vi "Generator PBP.vi"(6 "Faza":dbl, 7 "Numeric":dbl, 8 "Offset":dbl, 9 "Czestotliwosc":dbl, 10 "Amplituda":dbl, 11 "Sygnal":T1(ring)) -> (3 "Wyjscie":dbl)   [LabVIEW 2019]
uses:
  <vilib>/ptbypt/NI_PtbyPt.lvlib
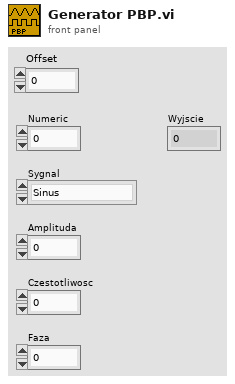
[diagram p1: front panel]
types:
  T1 = enum16{"Sinus", "Prostokąt", "Piła", "Trójkąt", "Rozkład losowy", "Rozkład normalny"}
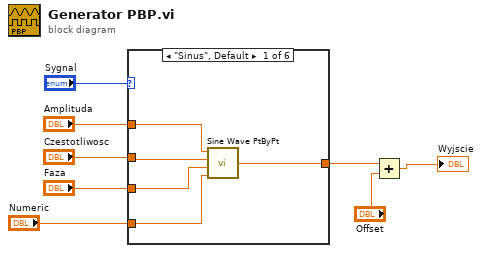
[diagram p0: block diagram]
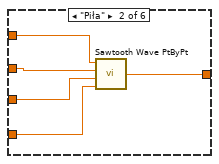
[diagram p2: hidden frame]
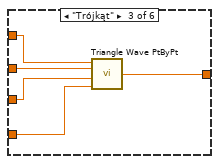
[diagram p3: hidden frame]
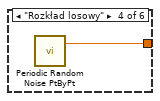
[diagram p4: hidden frame]
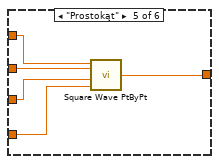
[diagram p5: hidden frame]
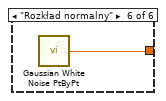
[diagram p6: hidden frame]
diagram:
  n1 = case shown="\"Sinus\", Default" "Sygnal" {
    tunnel: "Amplituda" -> [w13 w15 w19 _ w25 _]
    tunnel: "Czestotliwosc" -> [w12 w16 w20 _ w26 _]
    tunnel: "Faza" -> [w11 w18 w21 _ w27 _]
    tunnel: "Numeric" -> [w10 w17 w22 _ w28 _]
    tunnel: [w9 w14 w23 w24 w29 w30] -> w3
    frame "Sinus", Default {
      n2 = call <vilib>:"Sine Wave PtByPt.vi"("time"=w10, "phase"=w11, "frequency"=w12, "amplitude"=w13) -> ("sine wave"=w9:dbl)
    }
    frame "Piła" {
      n3 = call <vilib>:"Sawtooth Wave PtByPt.vi"("time"=w17, "phase"=w18, "frequency"=w16, "amplitude"=w15) -> ("sawtooth wave"=w14:dbl)
    }
    frame "Trójkąt" {
      n4 = call <vilib>:"Triangle Wave PtByPt.vi"("time"=w22, "phase"=w21, "frequency"=w20, "amplitude"=w19) -> ("triangle wave"=w23:dbl)
    }
    frame "Rozkład losowy" {
      n5 = call <vilib>:"Periodic Random Noise PtByPt.vi"() -> ("periodic random noise"=w24:dbl)  [unwired: 4 in, 1 out]
    }
    frame "Prostokąt" {
      n6 = call <vilib>:"Square Wave PtByPt.vi"("amplitude"=w25, "frequency"=w26, "phase"=w27, "time"=w28) -> ("square wave"=w29:dbl)  [unwired: 1 in]
    }
    frame "Rozkład normalny" {
      n7 = call <vilib>:"Gaussian White Noise PtByPt.vi"() -> ("Gaussian white noise"=w30:dbl)  [unwired: 3 in]
    }
  }
  n8 = Add(x=w3, y="Offset") -> (x+y=→"Wyjscie":dbl)
